vi "Andor_iXon_GetData_Point-Inttrace.vi"(8 "Input Cluster":T6, 10 "Cluster":T7, 11 "Measure":bool) -> (0 "Output Cluster":T6)   [LabVIEW 2009]
uses:
  atmcd32d.llb/AcquisitionMode_mode typedef.ctl
  atmcd32d.llb/ReadMode_mode typedef.ctl
  atmcd32d.llb/TriggerMode_mode typedef.ctl
  atmcd32d.llb/Shutter_type typedef.ctl
  atmcd32d.llb/Shutter_mode typedef.ctl
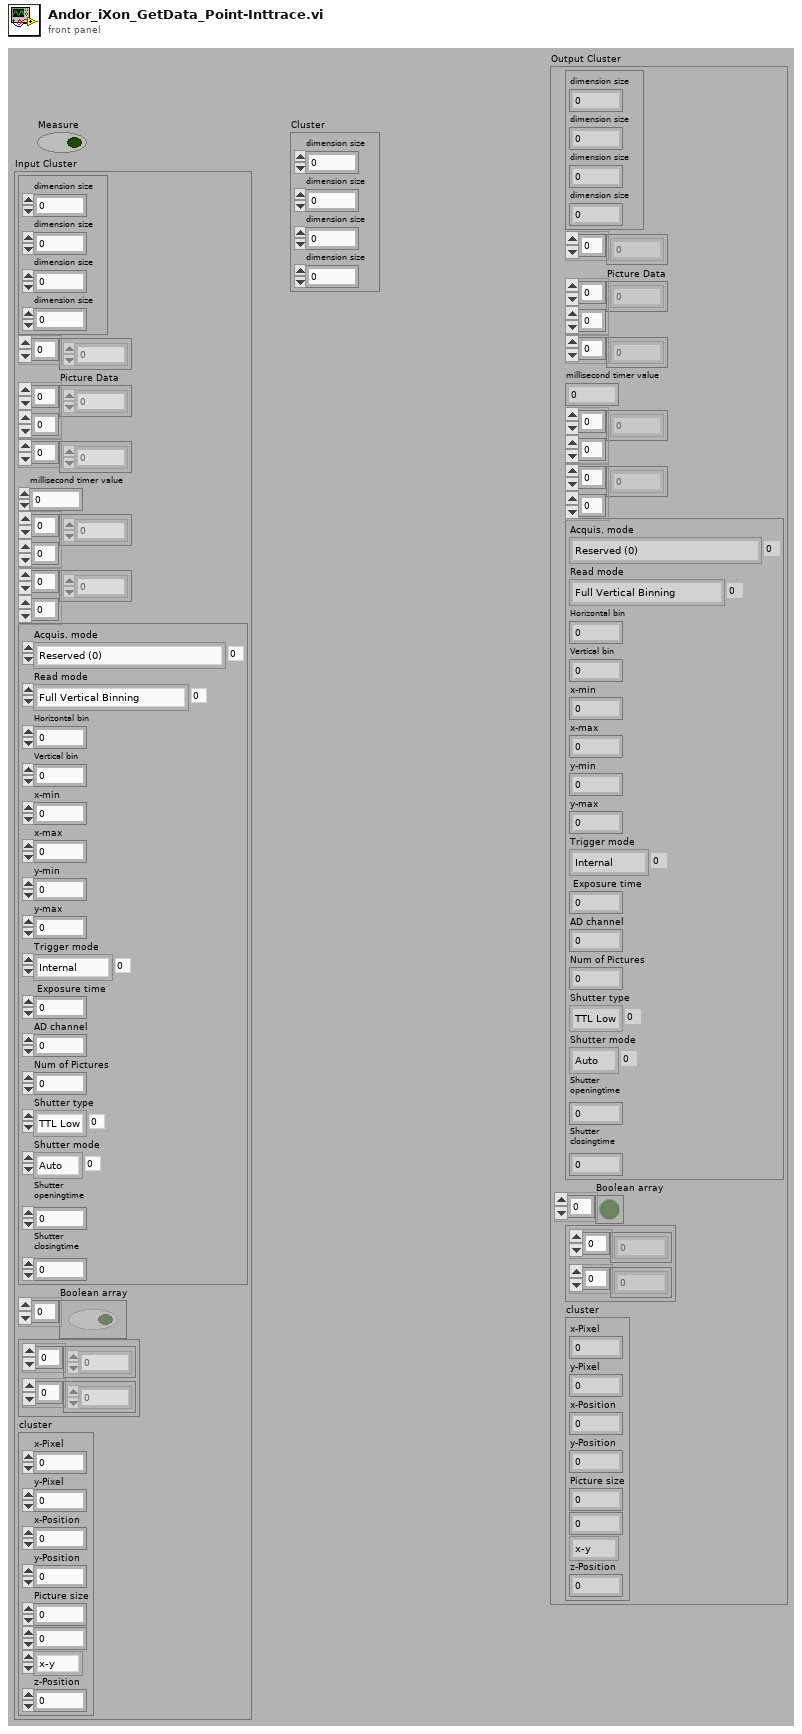
[diagram p1: front panel]
types:
  T1 = typedef "AcquisitionMode_mode typedef.ctl" = enum16{"Reserved (0)", "Single Scan", "Accumulate", "Kinetics", "Fast Kinetics", "Run Till Abort", "Reserved (6)", "Reserved (7)", "Reserved (8)", "Time Delayed Integration"}
  T2 = typedef "ReadMode_mode typedef.ctl" = enum16{"Full Vertical Binning", "Multi-Track", "Random-Track", "Single-Track", "Image"}
  T3 = typedef "TriggerMode_mode typedef.ctl" = enum16{"Internal", "External", "N/A (2)", "N/A (3)", "N/A (4)", "N/A (5)", "External Start"}
  T4 = typedef "Shutter_type typedef.ctl" = enum16{"TTL Low", "TTL High"}
  T5 = typedef "Shutter_mode typedef.ctl" = enum16{"Auto", "Open", "Close"}
  T6 = cluster{cluster{"dimension size":i32, "dimension size":i32, "dimension size":i32, "dimension size":i32}, i32[], "Picture Data":dbl[][], u32[], "millisecond timer value":u32, dbl[][], i32[][], cluster{"Acquis. mode":T1, "Read mode":T2, "Horizontal bin":i32, "Vertical bin":i32, "x-min":i32, "x-max":i32, "y-min":i32, "y-max":i32, "Trigger mode":T3, " Exposure time":sgl, "AD channel":i32, "Num of Pictures":i32, "Shutter type":T4, "Shutter mode":T5, "Shutter\nopeningtime":i32, "Shutter\nclosingtime":i32}, "Boolean array":bool[], cluster{dbl[], dbl[]}, "cluster":cluster{"x-Pixel":u16, "y-Pixel":u16, "x-Position":dbl, "y-Position":dbl, "Picture size":dbl, dbl, enum32{"x-y", "x-z", "y-z"}, "z-Position":dbl}}
  T7 = cluster{"dimension size":i32, "dimension size":i32, "dimension size":i32, "dimension size":i32}
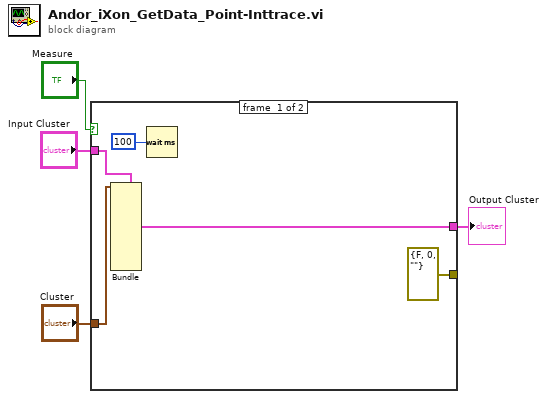
[diagram p0: block diagram]
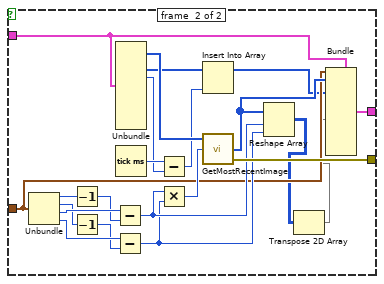
[diagram p2: hidden frame]
diagram:
  n1 = case shown="True" "Measure" {
    tunnel: [errorcluster {"status"=FALSE, "code"=0, "source"=""} ("error out") w31] -> _
    tunnel: "Cluster" -> [w7 w20]
    tunnel: "Input Cluster" -> [w5 w15]
    tunnel: [w6 w22] -> w2
    frame #0 {
      n2 = Bundle(cluster=w5, w7) -> (w6:T6)  [unwired: 10 out]
      n3 = Wait (ms)(milliseconds to wait=100) -> ()  [unwired: 1 out]
    }
    frame #1 {
      n4 = Unbundle(w20) -> ("dimension size"=w19:i32, "dimension size"=w17:i32, "dimension size"=w30:i32, "dimension size"=w29:i32)
      n5 = Decrement(x=w19) -> (x-1=w18:i32)
      n6 = Decrement(x=w17) -> (x-1=w16:i32)
      n7 = Subtract(x=w30, y=w18) -> (x-y=w26:i32)
      n8 = Subtract(x=w29, y=w16) -> (x-y=w25:i32)
      n9 = Unbundle(w15) -> (w24:i32[], w14:u32[], "millisecond timer value"=w21:u32)  [unwired: 8 out]
      n10 = Tick Count (ms)() -> (millisecond timer value=w27:u32)
      n11 = Subtract(x=w27, y=w21) -> (x-y=w13:u32)
      n12 = Multiply(x=w26, y=w25) -> (x*y=w28:i32)
      n13 = Insert Into Array "Insert Into Array"(array=w14, new element=w13) -> (w12:u32[])  [unwired: 1 in]
      n14 = call "GetMostRecentImage.vi"("size"=w28, "array"=w24) -> ("error out"=w31:errorcluster, "array"=w23:i32[])  [unwired: 1 in, 1 out]
      n15 = Reshape Array(w23, w26, w25) -> (w11:i32[][])
      n16 = Transpose 2D Array(2D array=w11) -> (transposed array=w10:i32[][])
      n17 = Bundle(cluster=w15, w20, w23, w12, w10) -> (w22:T6)  [unwired: 7 out]
    }
  }
  "Output Cluster" <- w2
